vi "1 Button Dialog.vi"(7 "Title":string, 8 "error in (no error)":errorcluster, 10 "Button name (\"OK\")":string="OK", 11 "Dialog Message":string) -> (0 "error out":errorcluster, 2 "result":bool)   [LabVIEW 2018]
panel:
  in  "X Stop":bool
  in  "True Button":bool
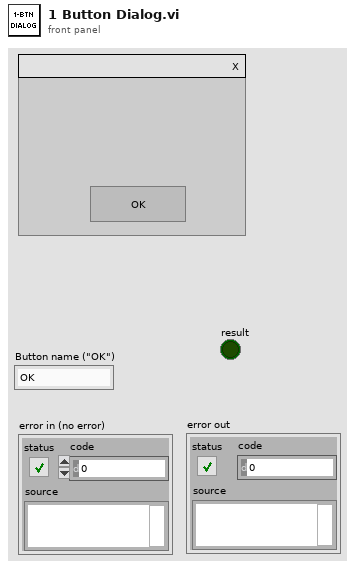
[diagram p1: front panel]
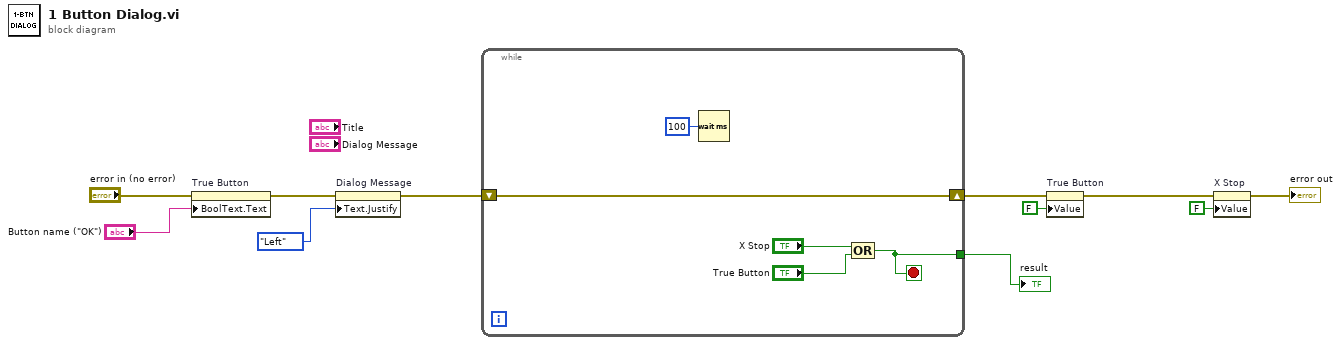
[diagram p0: block diagram]
diagram:
  n1 = property on="True Button" class="Bool (strict)"(error in="error in (no error)", "BoolText.Text"="Button name (\"OK\")") -> (error out=w2:errorcluster)  [unwired: 1 in, 1 out]
  n2 = property on="Dialog Message" class="Str"(error in=w2, "Text.Justify"=enum16{"Left", "Center", "Right"}."Left" ("Text.Justification")) -> (error out=w1:errorcluster)  [unwired: 1 in, 1 out]
  n3 = while {
    shift-right: [w16] -> w10
    shift-left: w1 -> [w16]
    tunnel: [w13] -> w6
    stop <- w13 stop-if-true
    n4 = Wait (ms)(milliseconds to wait=u32 100) -> ()  [unwired: 1 out]
    n5 = Compound Arithmetic op=OR("X Stop", "True Button") -> (w13:bool)
  }
  "result" <- w6
  n6 = property on="True Button" class="Bool (strict)"(error in=w10, "Value"=FALSE ("OK Button")) -> (error out=w7:errorcluster)  [unwired: 1 in, 1 out]
  n7 = property on="X Stop" class="Bool (strict)"(error in=w7, "Value"=FALSE ("OK Button")) -> (error out=→"error out":errorcluster)  [unwired: 1 in, 1 out]
